vi "4155C STOP flag.vi"() -> ()   [LabVIEW 2016]
doc: "Set to true to indicate an emergency stop. Reset to false before taking a measurement."
panel:
  in  "Emergency stop":bool
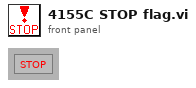
[diagram p1: front panel]
diagram:
